vi "command_generator.vi"(2 "commands":T1=enum."get acceleration", 3 "args":string[](array[string])) -> (16 "raw_command":string)   [LabVIEW 2012]
doc: "Each (raw) string command (some with optional parameters) detailed in the stepper motor control API documentation may be a little less than intuitive when developing a higher level application to control the hardware. This VI is designed to use an enumerated control of available commands (and an array of type String for any option parameters) and converts that input to the proper, formatted (raw) string command expected of the API.\n\nProduced By:\n\nChristopher Lemieux\nKod Integrations, LLC\n4835 Marianne Drive\nMount Airy, MD 21771\nhttp://www.kodintegrations.com\nemail: clemieux@kodintegrations.com\nphone: (240) 687-1288"
uses:
  commands.ctl
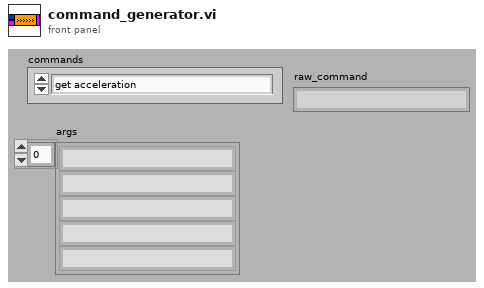
[diagram p1: front panel]
types:
  T1 = typedef "commands.ctl" = enum16{"clear error", "constant jog(-)", "constant jog(+)", "get acceleration", "get actual current", "get device id", "get digital input status", "get digial inputs status", "get dig output status", "get digital outputs status", "get firmware ver", "get high speed", "get idle current", "get low speed", "get micro step", "get motor status", "get move mode", "get polarity", "get position", "get product id", "get power status", "get run current", "get status", "home(-)", "home(+)", "move to position", "power down", "power up", "set acceleration", "set device id", "set digital output", "set digital outputs", "set high speed", "set idle current", "set low speed", "set move mode absolute", "set move mode increment", "set polarity", "set position", "set run current", "stop immediate", "stop slow", "store to memory"}
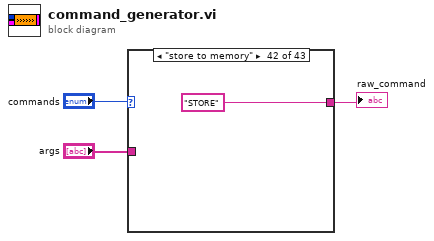
[diagram p0: block diagram]
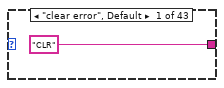
[diagram p2: hidden frame]
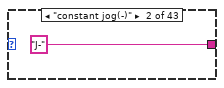
[diagram p3: hidden frame]
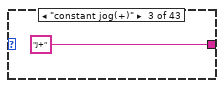
[diagram p4: hidden frame]
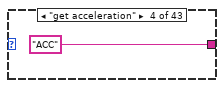
[diagram p5: hidden frame]
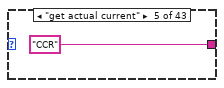
[diagram p6: hidden frame]
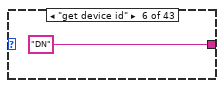
[diagram p7: hidden frame]
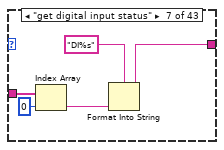
[diagram p8: hidden frame]
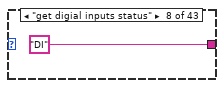
[diagram p9: hidden frame]
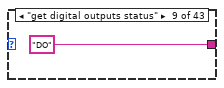
[diagram p10: hidden frame]
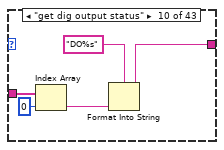
[diagram p11: hidden frame]
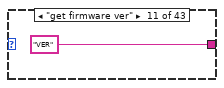
[diagram p12: hidden frame]
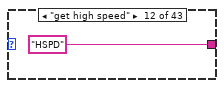
[diagram p13: hidden frame]
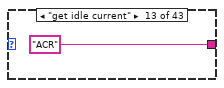
[diagram p14: hidden frame]
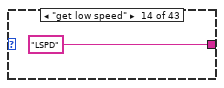
[diagram p15: hidden frame]
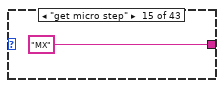
[diagram p16: hidden frame]
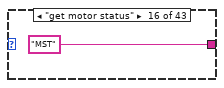
[diagram p17: hidden frame]
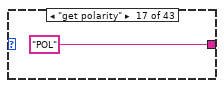
[diagram p18: hidden frame]
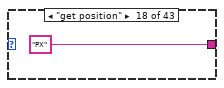
[diagram p19: hidden frame]
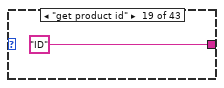
[diagram p20: hidden frame]
diagram:
  n1 = case shown="\"store to memory\"" "commands" {
    tunnel: ["CLR" "J-" "J+" "ACC" "CCR" "DN" w10 "DI" "DO" w17 "VER" "HSPD" "ACR" "LSPD" "MX" "MST" "POL" "PX" "ID" "EO" "CUR" "MST" "H-" "H+" w36 "EO=0" "EO=1" w43 w48 w53 w58 w63 w70 w75 "ABS" "INC" "MM" w83 w88 w93 "ABORT" "STORE" "STOP"] -> w2
    tunnel: "args" -> [_ _ _ _ _ _ w13 _ _ w20 _ _ _ _ _ _ _ _ _ _ _ _ _ _ w39 _ _ w46 w51 w56 w61 w66 w73 w78 _ _ _ w86 w91 w96 _ _ _]
    frame "clear error", Default {
    }
    frame "constant jog(-)" {
    }
    frame "constant jog(+)" {
    }
    frame "get acceleration" {
    }
    frame "get actual current" {
    }
    frame "get device id" {
    }
    frame "get digital input status" {
      n2 = Index Array(array=w13, index=0) -> (element=w11:string)
      n3 = Format Into String(format string="DI%s", w11) -> (resulting string=w10:string)  [unwired: 2 in, 1 out]
    }
    frame "get digial inputs status" {
    }
    frame "get digital outputs status" {
    }
    frame "get dig output status" {
      n4 = Index Array(array=w20, index=0) -> (element=w18:string)
      n5 = Format Into String(format string="DO%s", w18) -> (resulting string=w17:string)  [unwired: 2 in, 1 out]
    }
    frame "get firmware ver" {
    }
    frame "get high speed" {
    }
    frame "get idle current" {
    }
    frame "get low speed" {
    }
    frame "get micro step" {
    }
    frame "get motor status" {
    }
    frame "get polarity" {
    }
    frame "get position" {
    }
    frame "get product id" {
    }
    frame "get power status" {
    }
    frame "get run current" {
    }
    frame "get status" {
    }
    frame "home(-)" {
    }
    frame "home(+)" {
    }
    frame "move to position" {
      n6 = Index Array(array=w39, index=0) -> (element=w37:string)
      n7 = Format Into String(format string="X%s", w37) -> (resulting string=w36:string)  [unwired: 2 in, 1 out]
    }
    frame "power down" {
    }
    frame "power up" {
    }
    frame "set acceleration" {
      n8 = Index Array(array=w46, index=0) -> (element=w44:string)
      n9 = Format Into String(format string="ACC=%s", w44) -> (resulting string=w43:string)  [unwired: 2 in, 1 out]
    }
    frame "set device id" {
      n10 = Index Array(array=w51, index=0) -> (element=w49:string)
      n11 = Format Into String(format string="DN=%s", w49) -> (resulting string=w48:string)  [unwired: 2 in, 1 out]
    }
    frame "set high speed" {
      n12 = Index Array(array=w56, index=0) -> (element=w54:string)
      n13 = Format Into String(format string="HSPD=%s", w54) -> (resulting string=w53:string)  [unwired: 2 in, 1 out]
    }
    frame "set idle current" {
      n14 = Index Array(array=w61, index=0) -> (element=w59:string)
      n15 = Format Into String(format string="ACR=%s", w59) -> (resulting string=w58:string)  [unwired: 2 in, 1 out]
    }
    frame "set low speed" {
      n16 = Index Array(array=w66, index=0) -> (element=w64:string)
      n17 = Format Into String(format string="LSPD=%s", w64) -> (resulting string=w63:string)  [unwired: 2 in, 1 out]
    }
    frame "set digital output" {
      n18 = Index Array(array=w73, index #1=0 ("index"), index #2=1 ("index")) -> (element #1=w71:string, element #2=w68:string)
      n19 = Format Into String(format string="DO%s=%s", w71, w68) -> (resulting string=w70:string)  [unwired: 2 in, 1 out]
    }
    frame "set digital outputs" {
      n20 = Index Array(array=w78, index=0) -> (element=w76:string)
      n21 = Format Into String(format string="DO=%s", w76) -> (resulting string=w75:string)  [unwired: 2 in, 1 out]
    }
    frame "set move mode absolute" {
    }
    frame "set move mode increment" {
    }
    frame "get move mode" {
    }
    frame "set polarity" {
      n22 = Index Array(array=w86, index=0) -> (element=w84:string)
      n23 = Format Into String(format string="POL=%s", w84) -> (resulting string=w83:string)  [unwired: 2 in, 1 out]
    }
    frame "set position" {
      n24 = Index Array(array=w91, index=0) -> (element=w89:string)
      n25 = Format Into String(format string="PX=%s", w89) -> (resulting string=w88:string)  [unwired: 2 in, 1 out]
    }
    frame "set run current" {
      n26 = Index Array(array=w96, index=0) -> (element=w94:string)
      n27 = Format Into String(format string="CUR=%s", w94) -> (resulting string=w93:string)  [unwired: 2 in, 1 out]
    }
    frame "stop immediate" {
    }
    frame "store to memory" {
    }
    frame "stop slow" {
    }
  }
  "raw_command" <- w2
